vi "Check Raster Point In Range.vi"(11 "Projected Triangle":T1={"Point 1"={"x"=0.0, "y"=0.0}, "Point 2"={"x"=0.0, "y"=0.0}, "Point 3"={"x"=0.0, "y"=0.0}, "Fill Colour"=12517256, "Alpha"=0.0, "Alpha Blending Enabled"=FALSE, "Texture 1"={"x"=0.0, "y"=0.0}, "Texture 2"={"x"=0.0, "y"=0.0}, "Texture 3"={"x"=0.0, "y"=0.0}}) -> (3 "Keep":bool)   [LabVIEW 2022 SP3, in "3D.lvlib"]
uses:
  3D.lvlib
  Triangle 2D.ctl
  Point 2D.ctl
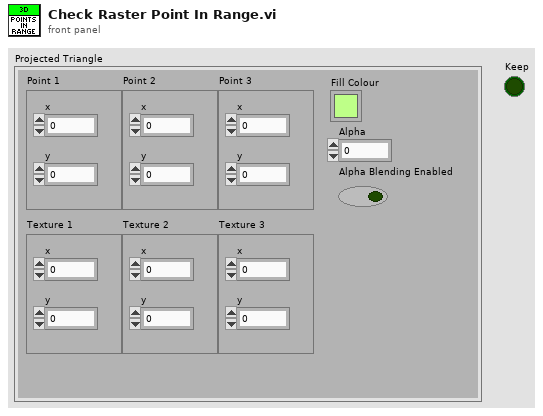
[diagram p1: front panel]
types:
  T1 = typedef "3D.lvlib/Triangle 2D.ctl" = cluster{"Point 1":T2, "Point 2":T2, "Point 3":T2, "Fill Colour":u32, "Alpha":dbl, "Alpha Blending Enabled":bool, "Texture 1":T2, "Texture 2":T2, "Texture 3":T2}
  T2 = typedef "3D.lvlib/Point 2D.ctl" = cluster{"x":sgl, "y":sgl}
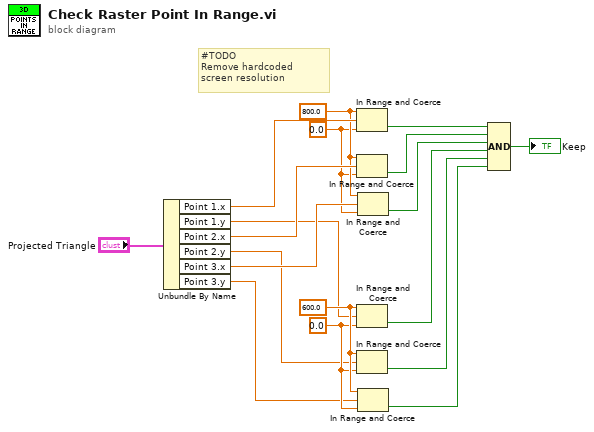
[diagram p0: block diagram]
diagram:
  w11 = sgl 0.0 ("lower limit")
  w12 = sgl 600.0 ("upper limit")
  w13 = sgl 0.0 ("lower limit")
  w14 = sgl 800.0 ("upper limit")
  # "#TODO\nRemove hardcoded screen resolution"
  n1 = Unbundle By Name("Projected Triangle") -> ("Point 1.x"=w17:sgl, "Point 1.y"=w10:sgl, "Point 2.x"=w16:sgl, "Point 2.y"=w9:sgl, "Point 3.x"=w15:sgl, "Point 3.y"=w8:sgl)
  n2 = In Range and Coerce(upper limit=w14, x=w17, lower limit=w13) -> (In Range?=w7:bool)  [unwired: 1 out]
  n3 = In Range and Coerce(upper limit=w14, x=w16, lower limit=w13) -> (In Range?=w6:bool)  [unwired: 1 out]
  n4 = In Range and Coerce(upper limit=w12, x=w10, lower limit=w11) -> (In Range?=w4:bool)  [unwired: 1 out]
  n5 = In Range and Coerce(upper limit=w12, x=w9, lower limit=w11) -> (In Range?=w3:bool)  [unwired: 1 out]
  n6 = In Range and Coerce(upper limit=w14, x=w15, lower limit=w13) -> (In Range?=w5:bool)  [unwired: 1 out]
  n7 = In Range and Coerce(upper limit=w12, x=w8, lower limit=w11) -> (In Range?=w2:bool)  [unwired: 1 out]
  n8 = Compound Arithmetic op=AND(w7, w6, w5, w4, w3, w2) -> (→"Keep":bool)
